vi "WBRT Init.vi"(8 "error in":errorcluster, 11 "WBRT State In":T1={"Encoders"={"Roll"=0.0, "Pitch"=0.0, "Yaw"=0.0, "Roll Trim"=0.0, "Pitch Trim"=0.0, "Yaw Trim"=0.0, "Roll Rate"=0.0, "Pitch Rate"=0.0, "Yaw Rate"=0.0}, "SPI Data"={"X-Gyro"=0.0, "Y-Gyro"=0.0, "Z-Gyro"=0.0, "X-Accel"=0.0, "Y-Accel"=0.0, "Z-Accel"=0.0}, "Camera"={"Numeric"=0.0}, "Filter Data"={"Filter Enabled?"=FALSE, "Filter Type"=enum."Equi-Ripple", "Pass Frequency"=1.0, "Stop Frequency (Equi-Ripple)"=0.45000000000000007, "Order"=0, "Ripple (dB)"=2.0}, "FPGA VI Reference"=refnum, "dt"=0.0, "Elapsed Time (msec)"=0, "Setpoints"={"Roll Setpoint (degrees)"=125.0, "Pitch Setpoint (degrees)"=125.0, "Yaw Setpoint (degrees)"=125.0}, "Commands"={"Left Command"=0.0, "Right Command"=0.0}, "Trajectory Data"=[], "Gains"={"Gain1"=0.0, "Gain2"=0.0, "Gain3"=0.0, "Gain4"=0.0, "Gain5"=0.0, "Gain6"=0.0, "Gain7"=0.0, "Gain8"=0.0, "Gain9"=0.0}, "Global Variables"={"Variable1"=[], "Variable2"=[], "Variable3"=[], "Variable4"=[]}, "Centroid"={"X Centroid"=0.0, "Y Centroid"=0.0}, "Error1"=0.0, "Error2"=0.0, "Error3"=0.0, "Error4"=0.0, "Recorded Data"=[], "Landing Factor"=0.0} {"Trajectory Data" format="%0.3f"; "Filter Data"."Stop Frequency (Equi-Ripple)" format="%0.3f"; "Filter Data"."Pass Frequency" format="%0.3f"}) -> (0 "error out":errorcluster, 3 "WBRT State Out":T1={"Encoders"={"Roll"=0.0, "Pitch"=0.0, "Yaw"=0.0, "Roll Trim"=0.0, "Pitch Trim"=0.0, "Yaw Trim"=0.0, "Roll Rate"=0.0, "Pitch Rate"=0.0, "Yaw Rate"=0.0}, "SPI Data"={"X-Gyro"=0.0, "Y-Gyro"=0.0, "Z-Gyro"=0.0, "X-Accel"=0.0, "Y-Accel"=0.0, "Z-Accel"=0.0}, "Camera"={"Numeric"=0.0}, "Filter Data"={"Filter Enabled?"=FALSE, "Filter Type"=enum."Equi-Ripple", "Pass Frequency"=1.0, "Stop Frequency (Equi-Ripple)"=0.45000000000000007, "Order"=0, "Ripple (dB)"=2.0}, "FPGA VI Reference"=refnum, "dt"=0.0, "Elapsed Time (msec)"=0, "Setpoints"={"Roll Setpoint (degrees)"=125.0, "Pitch Setpoint (degrees)"=125.0, "Yaw Setpoint (degrees)"=125.0}, "Commands"={"Left Command"=0.0, "Right Command"=0.0}, "Trajectory Data"=[], "Gains"={"Gain1"=0.0, "Gain2"=0.0, "Gain3"=0.0, "Gain4"=0.0, "Gain5"=0.0, "Gain6"=0.0, "Gain7"=0.0, "Gain8"=0.0, "Gain9"=0.0}, "Global Variables"={"Variable1"=[], "Variable2"=[], "Variable3"=[], "Variable4"=[]}, "Centroid"={"X Centroid"=0.0, "Y Centroid"=0.0}, "Error1"=0.0, "Error2"=0.0, "Error3"=0.0, "Error4"=0.0, "Recorded Data"=[], "Landing Factor"=0.0} {"Trajectory Data" format="%0.3f"; "Filter Data"."Stop Frequency (Equi-Ripple)" format="%0.3f"; "Filter Data"."Pass Frequency" format="%0.3f"})   [LabVIEW 2012]
doc: "Initializes the WBRT code. This reads in any trajectory data and trim data, and initializes the FPGA driver.\n\nAuthor: Brandon Steele\n\nCopyright: Brigham Young University"
uses:
  Custom Controls/WBRT State.ctl
  Custom Controls/WBRT Encoders.ctl
  Custom Controls/WBRT SPI Data.ctl
  Custom Controls/WBRT Filter Data.ctl
  Custom Controls/WBRT Filter Type.ctl
  FPGA Samples/spi_single port_example/Host API/Controls/FPGA SPI_FPGA Ref.ctl
  Custom Controls/WBRT Setpoints.ctl
  Custom Controls/WBRT Commands.ctl
  Custom Controls/WBRT Gains.ctl
  Custom Controls/WBRT Global Variables.ctl
  FPGA Samples/spi_single port_example/Host API/Controls/FPGA SPI_SPI Configuration Cluster.ctl
  <vilib>/FPGAPlugInAG/cRIO-9111/niLvFpga_Open_cRIO-9111.vi
  <vilib>/Utility/error.llb/Error Cluster From Error Code.vi
  <vilib>/rvi/errors/niLvFpgaAdjustHostInterfaceError.vi
  <vilib>/rvi/interface/nirviOpenFPGA/nirviOpenFPGA.xnode
  FPGA Bitfiles/Whirlybird_FPGATarget_WhirlybirdFPGAMa_DBA2D843.lvbitx
  Whirlybird FPGA Main.vi
  <vilib>/rvi/interface/nirviReadWriteControl/nirviReadWriteControl.xnode
  NiFpgaLv.dll
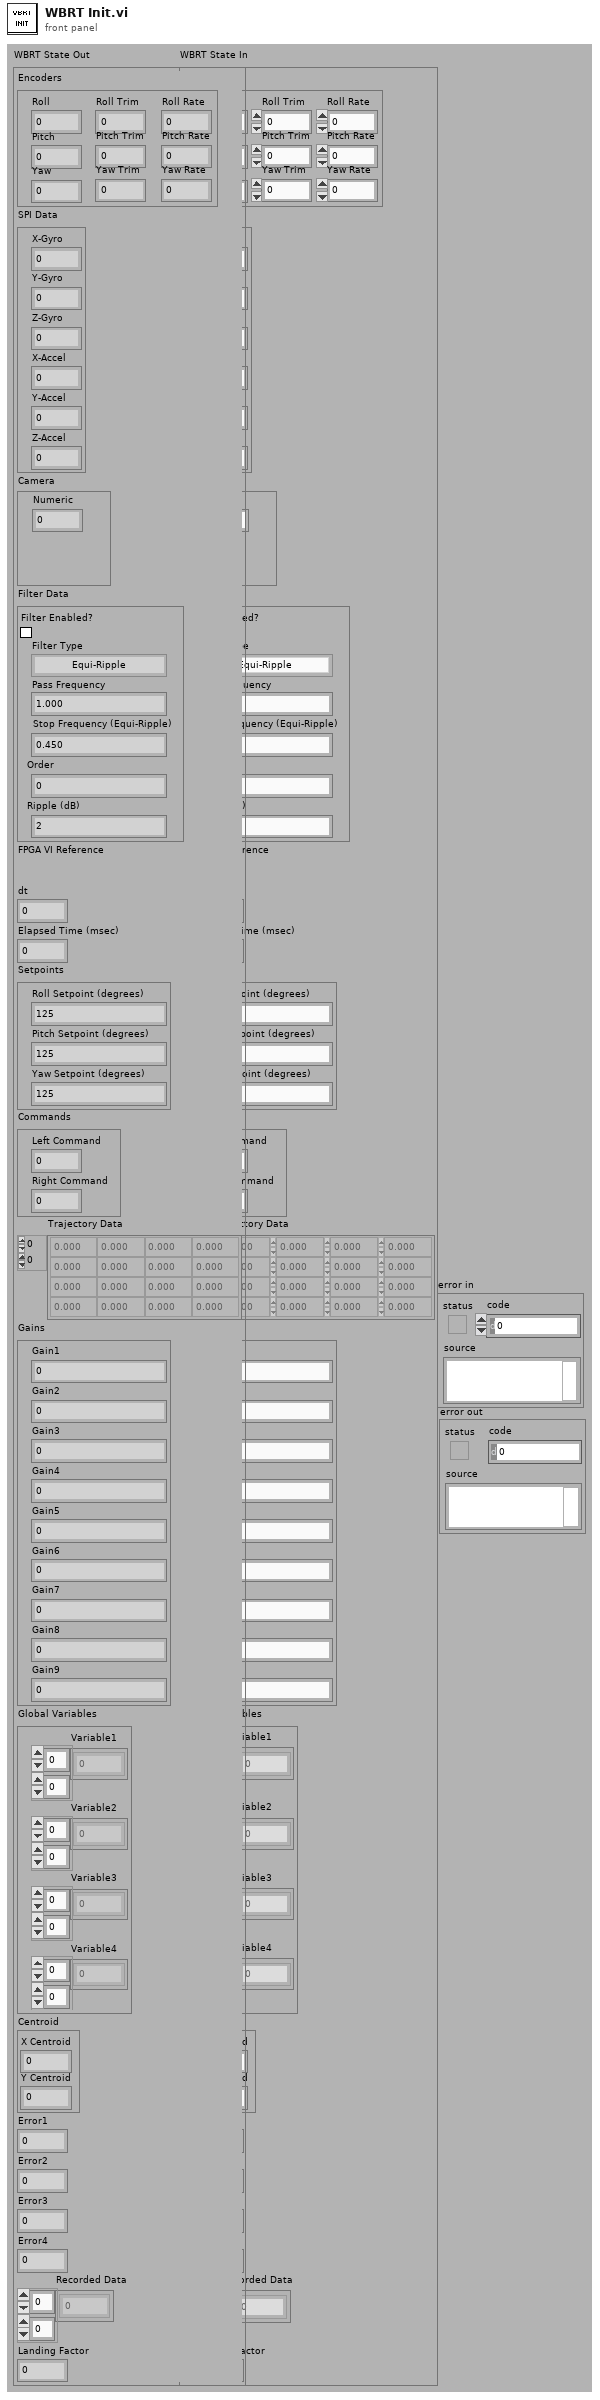
[diagram p1: front panel]
types:
  T1 = typedef "WBRT State.ctl" = cluster{"Encoders":T2, "SPI Data":T3, "Camera":cluster{"Numeric":dbl}, "Filter Data":T4, "FPGA VI Reference":T6, "dt":dbl, "Elapsed Time (msec)":u32, "Setpoints":T7, "Commands":T8, "Trajectory Data":dbl[][], "Gains":T9, "Global Variables":T10, "Centroid":cluster{"X Centroid":sgl, "Y Centroid":sgl}, "Error1":dbl, "Error2":dbl, "Error3":dbl, "Error4":dbl, "Recorded Data":dbl[][], "Landing Factor":dbl}
  T2 = typedef "WBRT Encoders.ctl" = cluster{"Roll":dbl, "Pitch":dbl, "Yaw":dbl, "Roll Trim":dbl, "Pitch Trim":dbl, "Yaw Trim":dbl, "Roll Rate":dbl, "Pitch Rate":dbl, "Yaw Rate":dbl}
  T3 = typedef "WBRT SPI Data.ctl" = cluster{"X-Gyro":dbl, "Y-Gyro":dbl, "Z-Gyro":dbl, "X-Accel":dbl, "Y-Accel":dbl, "Z-Accel":dbl}
  T4 = typedef "WBRT Filter Data.ctl" = cluster{"Filter Enabled?":bool, "Filter Type":T5, "Pass Frequency":dbl, "Stop Frequency (Equi-Ripple)":dbl, "Order":i32, "Ripple (dB)":dbl}
  T5 = typedef "WBRT Filter Type.ctl" = enum16{"Equi-Ripple", "Butterworth", "Chebyshev"}
  T6 = typedef "FPGA SPI_FPGA Ref.ctl" = refnum<k20>
  T7 = typedef "WBRT Setpoints.ctl" = cluster{"Roll Setpoint (degrees)":dbl, "Pitch Setpoint (degrees)":dbl, "Yaw Setpoint (degrees)":dbl}
  T8 = typedef "WBRT Commands.ctl" = cluster{"Left Command":dbl, "Right Command":dbl}
  T9 = typedef "WBRT Gains.ctl" = cluster{"Gain1":dbl, "Gain2":dbl, "Gain3":dbl, "Gain4":dbl, "Gain5":dbl, "Gain6":dbl, "Gain7":dbl, "Gain8":dbl, "Gain9":dbl}
  T10 = typedef "WBRT Global Variables.ctl" = cluster{"Variable1":dbl[][], "Variable2":dbl[][], "Variable3":dbl[][], "Variable4":dbl[][]}
  T11 = typedef "FPGA SPI_SPI Configuration Cluster.ctl" = cluster{"CS":u8, "Clock Rate (Hz)":dbl, "Clock Mode":u8, "CS Active State":bool}
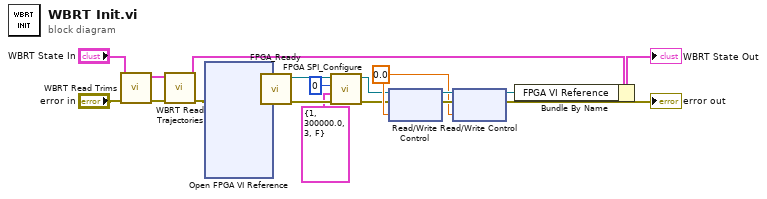
[diagram p0: block diagram]
diagram:
  w9 = 0.0 ("CommandA")
  n1 = call "WBRT Read Trims.vi"("error in"="error in", "WBRT State In"="WBRT State In") -> ("error out"=w4:errorcluster, "WBRT State Out"=w2:T1)  [unwired: 8 in]
  n2 = call "WBRT Read Trajectories.vi"("error in"=w4, "WBRT State In"=w2) -> ("error out"=w3:errorcluster, "WBRT State Out"=w1:T1)  [unwired: 8 in]
  n3 = xnode "Open FPGA VI Reference"("error in"=w3) -> ("FPGA VI Reference Out"=w15:T6, "error out"=w20:errorcluster)  [unwired: 1 in]
  n4 = call "FPGA_Ready.vi"("Error In"=w20, "FPGA VI Reference In"=w15) -> ("Error Out"=w18:errorcluster, "FPGA VI Reference Out"=w17:T6)  [unwired: 7 out]
  n5 = call "FPGA SPI_Configure.vi"("error in"=w18, "Configuration Cluster"=T11 {"CS"=1, "Clock Rate (Hz)"=300000.0, "Clock Mode"=3, "CS Active State"=FALSE} ("SPI Configuration Cluster"), "Port"=u8 0, "FPGA VI Reference"=w17) -> ("error out"=w8:errorcluster, "FPGA VI Reference Out"=w7:T6)  [unwired: 5 in, 1 out]
  n6 = xnode "Read/Write Control"("FPGA VI Reference In"=w7, "error in"=w8, "MC2"=w9) -> ("FPGA VI Reference Out"=w11:T6, "error out"=w10:errorcluster)
  n7 = xnode "Read/Write Control"("FPGA VI Reference In"=w11, "error in"=w10, "MC1"=w9) -> ("FPGA VI Reference Out"=w5:T6, "error out"=→"error out":errorcluster)
  n8 = Bundle By Name(cluster=w1, "FPGA VI Reference"=w5) -> (→"WBRT State Out":T1)
